vi "Transfer LSS Real.vi"(1 "precision":u32, 2 "lambda":cdb[](array[numeric]) format="%.2f", 3 "beta":dbl[](array[numeric]) format="%.2f") -> (0 "formula linear combination":string)   [LabVIEW 2010, in "NI_Gmath.lvlib"]
uses:
  NI_Gmath.lvlib
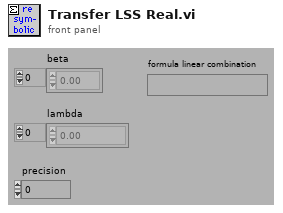
[diagram p1: front panel]
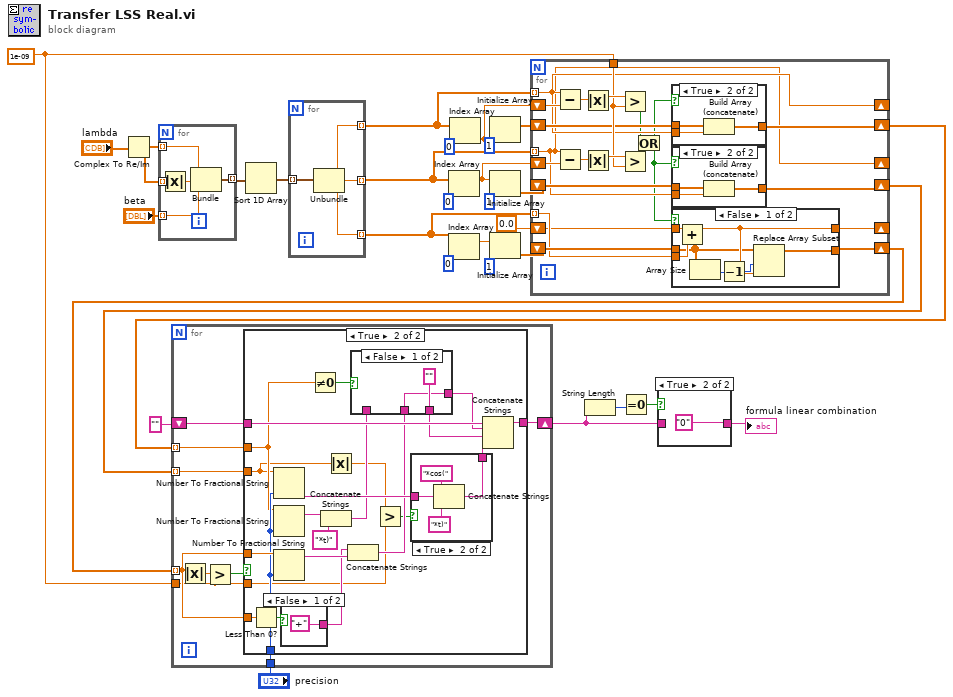
[diagram p0: block diagram]
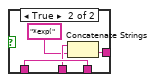
[diagram p4: hidden frame]
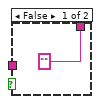
[diagram p5: hidden frame]
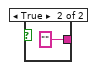
[diagram p6: hidden frame]
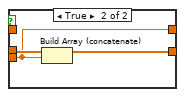
[diagram p7: hidden frame]
diagram:
  w1 = 1e-09
  n1 = Complex To Re/Im(x + iy="lambda") -> (x=w29:dbl[], y=w28:dbl[])
  n2 = for {
    tunnel: w29 -> [w37] mode=indexing
    tunnel: w28 -> [w36] mode=indexing
    tunnel: "beta" -> [w35] mode=indexing
    tunnel: [w34] -> w30 mode=indexing
    n3 = Absolute Value(x=w36) -> (abs(x)=w33:dbl)
    n4 = Bundle(w37, w33, w35) -> (w34:cluster{dbl, dbl, dbl})  [unwired: 1 in]
  }
  n5 = Sort 1D Array(array=w30) -> (sorted array=w27:cluster{dbl, dbl, dbl}[])
  n6 = for {
    tunnel: w27 -> [w41] mode=indexing
    tunnel: [w40] -> w15 mode=indexing
    tunnel: [w39] -> w14 mode=indexing
    tunnel: [w38] -> w13 mode=indexing
    n7 = Unbundle(w41) -> (w40:dbl, w39:dbl, w38:dbl)
  }
  n8 = Index Array(array=w14, index=0) -> (element=w16:dbl)
  n9 = Index Array(array=w13, index=0) -> (element=w10:dbl)
  n10 = Index Array(array=w15, index=0) -> (element=w17:dbl)
  n11 = Initialize Array(w17, 1) -> (w23:dbl[])
  n12 = Initialize Array(w16, 1) -> (w22:dbl[])
  n13 = Initialize Array(w10, 1) -> (w21:dbl[])
  n14 = for {
    shift-right: [w54] -> w12
    shift-left: w23 -> [w55]
    shift-right: [w52] -> w11
    shift-left: w22 -> [w53]
    shift-right: [w50] -> w3
    shift-left: w21 -> [w51]
    shift-right: [w48] -> _
    shift-left: w17 -> [w62]
    shift-right: [w47] -> _
    shift-left: w16 -> [w56]
    tunnel: w15 -> [w48] mode=indexing
    tunnel: w1 -> [w57]
    tunnel: w14 -> [w47] mode=indexing
    tunnel: w13 -> [w49] mode=indexing
    shift-right: [w43] -> _
    shift-left: 0.0 -> [w44]
    n15 = Subtract(x=w48, y=w62) -> (x-y=w61:dbl)
    n16 = Subtract(x=w47, y=w56) -> (x-y=w58:dbl)
    n17 = Absolute Value(x=w61) -> (abs(x)=w60:dbl)
    n18 = Absolute Value(x=w58) -> (abs(x)=w59:dbl)
    n19 = Greater?(x=w60, y=w57) -> (0:w46:bool)
    n20 = Greater?(x=w59, y=w57) -> (0:w45:bool)
    n21 = Or(x=w46, y=w45) -> (x .or. y?=w42:bool)
    n22 = case shown="True" w42 {
      tunnel: w55 -> [w77 w80]
      tunnel: [w77 w79] -> w54
      tunnel: w48 -> [_ w78]
      frame False {
      }
      frame True {
        n23 = Build Array (concatenate)(w80, w78) -> (w79:dbl[])
      }
    }
    n24 = case shown="True" w42 {
      tunnel: w53 -> [w73 w76]
      tunnel: [w73 w75] -> w52
      tunnel: w47 -> [_ w74]
      frame False {
      }
      frame True {
        n25 = Build Array (concatenate)(w76, w74) -> (w75:dbl[])
      }
    }
    n26 = case shown="False" w42 {
      tunnel: w51 -> [w65 w72]
      tunnel: [w66 w71] -> w50
      tunnel: w49 -> [w68 w70]
      tunnel: w44 -> [w69 _]
      tunnel: [w67 w70] -> w43
      frame False {
        n27 = Add(x=w69, y=w68) -> (x+y=w67:dbl)
        n28 = Array Size(array=w65) -> (size(s)=w64:i32)
        n29 = Decrement(x=w64) -> (x-1=w63:i32)
        n30 = Replace Array Subset(array=w65, new element=w67, index=w63) -> (w66:dbl[])
      }
      frame True {
        n31 = Build Array (concatenate)(w72, w70) -> (w71:dbl[])
      }
    }
  }
  n32 = for {
    shift-right: [w86] -> w6
    shift-left: "" -> [w87]
    tunnel: w3 -> [w84] mode=indexing
    tunnel: "precision" -> [w89]
    tunnel: w12 -> [w88] mode=indexing
    tunnel: w11 -> [w85] mode=indexing
    tunnel: w1 -> [w81]
    n33 = Absolute Value(x=w84) -> (abs(x)=w83:dbl)
    n34 = Greater?(x=w83, y=w81) -> (0:w82:bool)
    n35 = case shown="True" w82 {
      tunnel: w89 -> [_ w104]
      tunnel: w84 -> [_ w112]
      tunnel: w88 -> [_ w100]
      tunnel: w87 -> [w90 w108]
      tunnel: [w90 w107] -> w86
      tunnel: w85 -> [_ w94]
      tunnel: w84 -> [_ w103]
      tunnel: w81 -> [_ w91]
      frame False {
      }
      frame True {
        n36 = Less Than 0?(x=w103) -> (x < 0?=w102:bool)
        n37 = Number To Fractional String(number=w94, precision (6)=w104) -> (F-format string=w106:string)  [unwired: 2 in]
        n38 = Number To Fractional String(number=w100, precision (6)=w104) -> (F-format string=w110:string)  [unwired: 2 in]
        n39 = Number To Fractional String(number=w112, precision (6)=w104) -> (F-format string=w111:string)  [unwired: 2 in]
        n40 = case shown="False" w102 {
          tunnel: ["+" ""] -> w101
          frame False {
          }
          frame True {
          }
        }
        n41 = Not Equal To 0?(x=w100) -> (x != 0?=w99:bool)
        n42 = Concatenate Strings(w110, "*t)") -> (w95:string)
        n43 = Absolute Value(x=w94) -> (abs(x)=w93:dbl)
        n44 = Concatenate Strings(w101, w111) -> (w98:string)
        n45 = case shown="False" w99 {
          tunnel: w98 -> [w113 w117]
          tunnel: [w113 w115] -> w97
          tunnel: ["" w118] -> w96
          tunnel: w95 -> [_ w118]
          frame False {
          }
          frame True {
            n46 = Concatenate Strings(w117, "*exp(") -> (w115:string)
          }
        }
        n47 = Greater?(x=w93, y=w91) -> (0:w92:bool)
        n48 = case shown="True" w92 {
          tunnel: ["" w121] -> w105
          tunnel: w106 -> [_ w120]
          frame False {
          }
          frame True {
            n49 = Concatenate Strings("*cos(", w120, "*t)") -> (w121:string)
          }
        }
        n50 = Concatenate Strings(w108, w97, w96, w105) -> (w107:string)
      }
    }
  }
  n51 = String Length(string=w6) -> (length=w5:i32)
  n52 = Equal To 0?(x=w5) -> (x = 0?=w4:bool)
  n53 = case shown="True" w4 {
    tunnel: w6 -> [w126 _]
    tunnel: [w126 "0"] -> w2
    frame False {
    }
    frame True {
    }
  }
  "formula linear combination" <- w2
